vi "Test99.vi"(7 "L2T":T1 caption="Limites de test pris en compte", 8 "errin":errorcluster, 9 "SN":string="0B5MEVA000CA1JC1M0000041", 10 "OCV":string) -> (0 "errout":errorcluster, 2 "chaîne concaténée":string)   [LabVIEW 2020]
uses:
  <userlib>/Sylvain.lib/DATA_INSERT.vi
  VarGLO/Global var.vi
  Ctrl/L2T.ctl
panel:
  out "CMD":string
  in  "Cell 5 et 6":T2
  out "dataBDD":string[](array[string])
  in  "Cell 1 et 2":T2
  in  "Cell 3 et 4":T2
  out "Out":T3
  # "Pre DCIR_____________________________________"
  # "intra DCIR_____________________________________"
  # "Post DCIR_____________________________________"
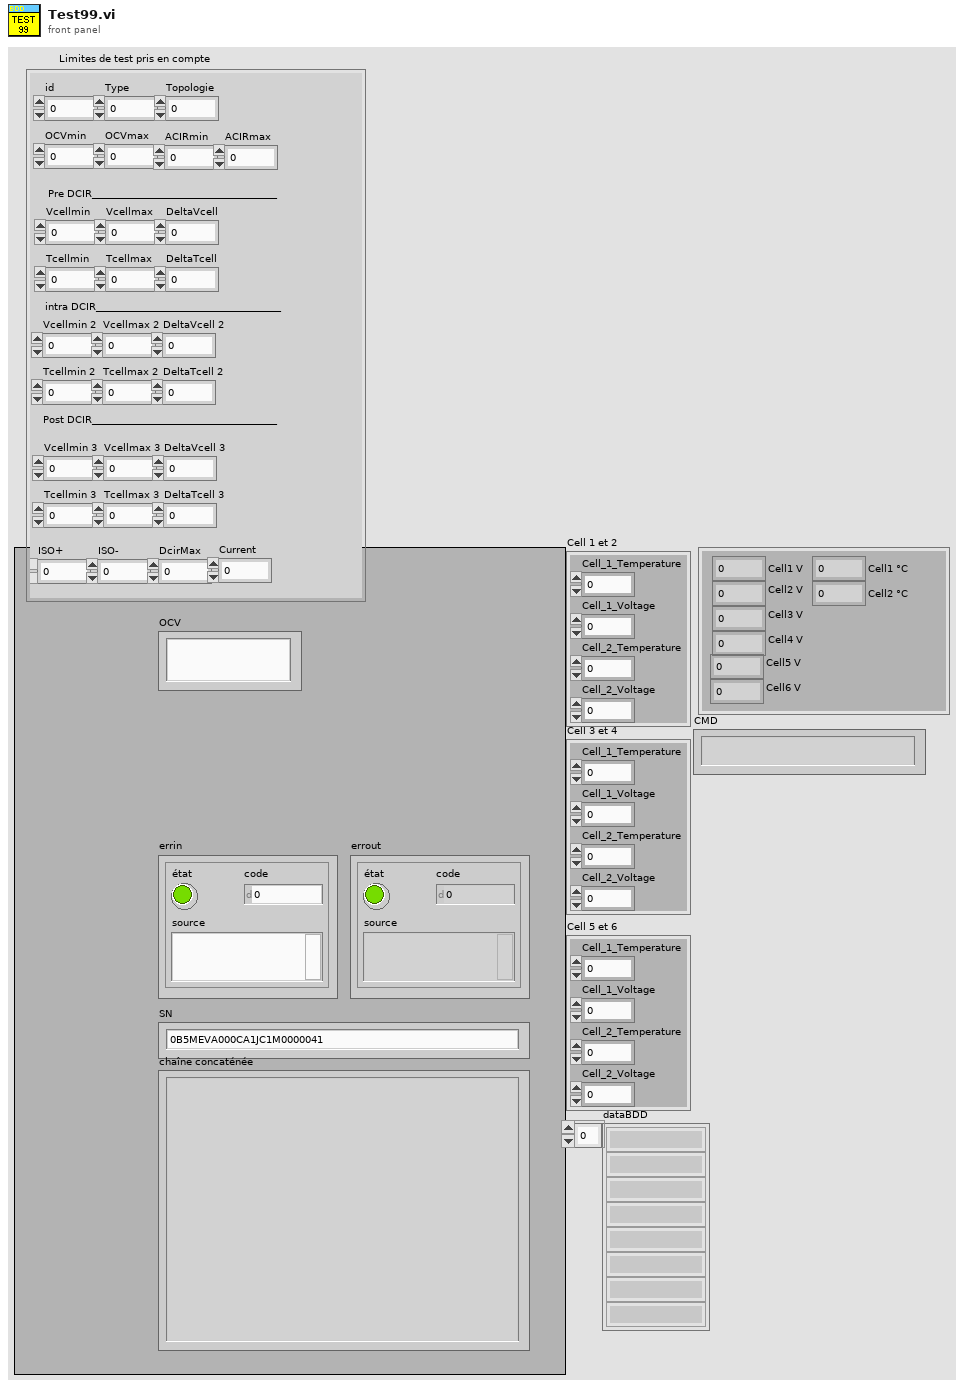
[diagram p1: front panel]
types:
  T1 = typedef "L2T.ctl" = cluster{"id":dbl, "Type":dbl, "OCVmin":dbl, "OCVmax":dbl, "ACIRmin":dbl, "ACIRmax":dbl, "Vcellmin":dbl, "Vcellmax":dbl, "DeltaVcell":dbl, "Tcellmin":dbl, "Tcellmax":dbl, "DeltaTcell":dbl, "ISO+":dbl, "ISO-":dbl, "DcirMax":dbl, "Current":dbl, "Topologie":dbl, "Vcellmin 2":dbl, "Vcellmax 2":dbl, "DeltaVcell 2":dbl, "Tcellmin 2":dbl, "Tcellmax 2":dbl, "DeltaTcell 2":dbl, "Vcellmin 3":dbl, "Vcellmax 3":dbl, "DeltaVcell 3":dbl, "Tcellmin 3":dbl, "Tcellmax 3":dbl, "DeltaTcell 3":dbl}
  T2 = cluster{"Cell_1_Temperature":sgl, "Cell_1_Voltage":sgl, "Cell_2_Temperature":sgl, "Cell_2_Voltage":sgl}
  T3 = cluster{"Cell1 V":sgl, "Cell2 V":sgl, "Cell3 V":sgl, "Cell4 V":sgl, "Cell1 °C":sgl, "Cell2 °C":sgl, "Cell5 V":sgl, "Cell6 V":sgl}
  T4 = cluster{"TempMin":sgl, "TempMax":sgl, "VoltageMin":sgl, "VoltageMax":sgl, "DeltaV":sgl, "DeltaC":sgl, "Ton":sgl}
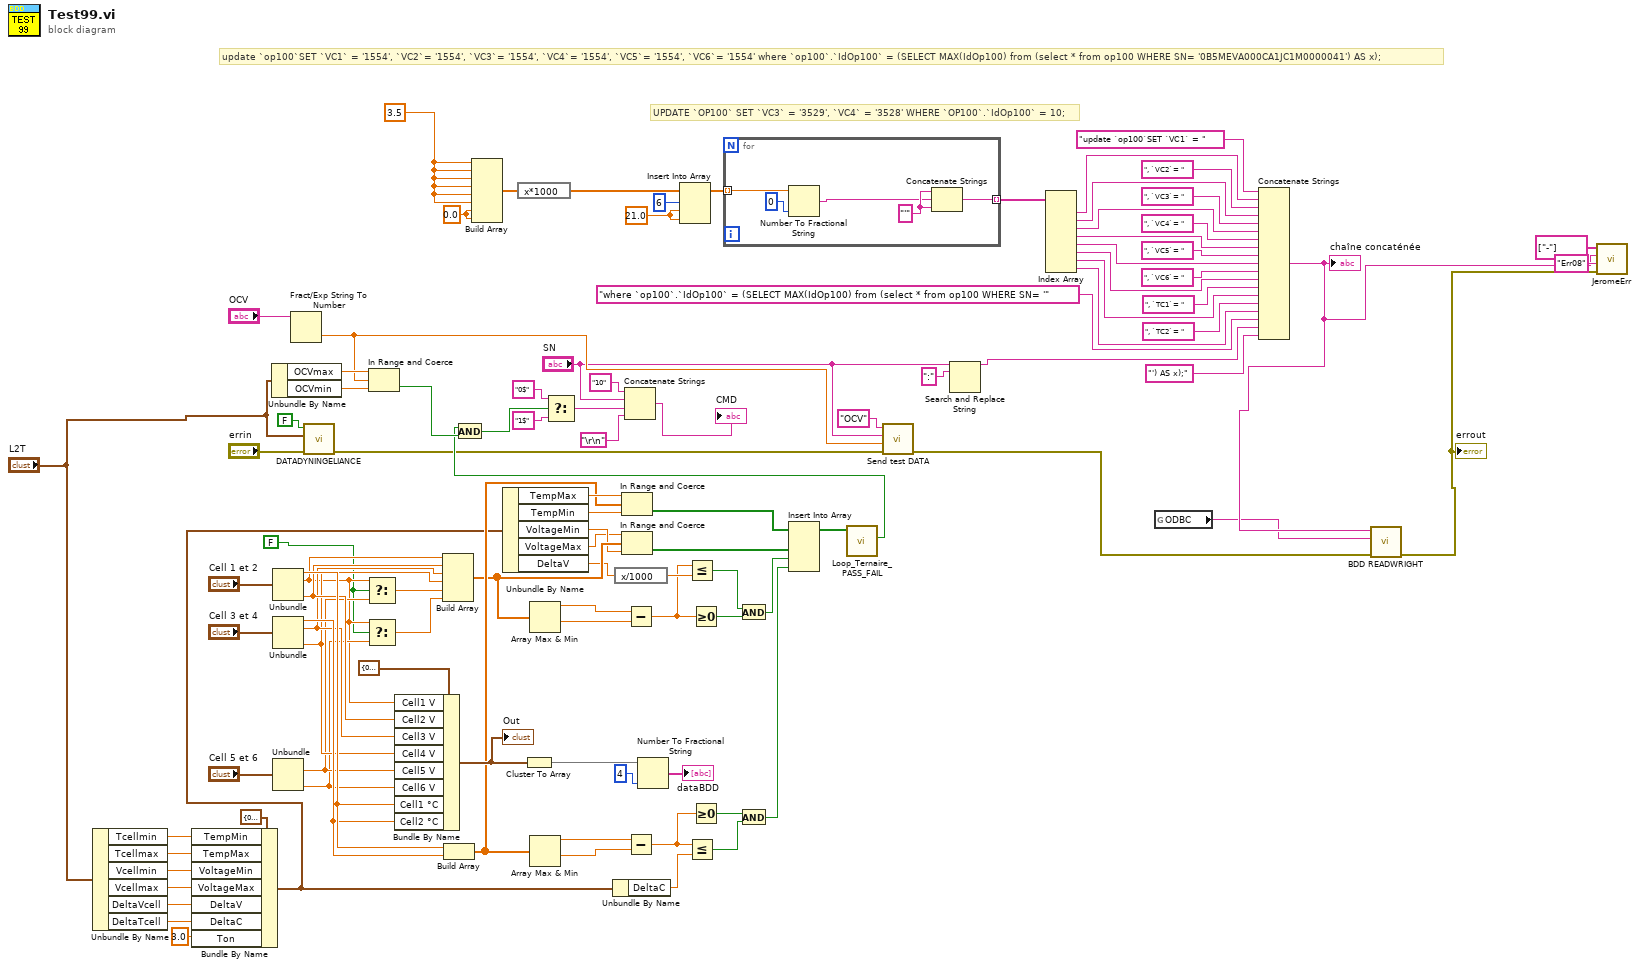
[diagram p0: block diagram]
diagram:
  w19 = FALSE ("sélecteur")
  w62 = sgl 21.0 ("nouvel élément/sous-tableau")
  w63 = sgl 3.5 ("élément")
  w99 = sgl 0.0 ("élément")
  # "update `op100`SET `VC1` = '1554', `VC2`= '1554', `VC3`= '1554', `VC4`= '1554', `VC5`= '1554', `VC6`= '1554' where `op100`.`IdOp100` = (SELECT MAX(IdOp100) from (select * from op100 WHERE SN= '0B5MEVA000CA1JC1M0000041') AS x);"
  # "UPDATE `OP100` SET `VC3` = '3529', `VC4` = '3528' WHERE `OP100`.`IdOp100` = 10;"
  n1 = Unbundle By Name("L2T") -> ("Tcellmin"=w17:dbl, "Tcellmax"=w16:dbl, "Vcellmin"=w15:dbl, "Vcellmax"=w14:dbl, "DeltaVcell"=w13:dbl, "DeltaTcell"=w12:dbl)
  n2 = Bundle By Name(cluster=T4 {"TempMin"=0.0, "TempMax"=0.0, "VoltageMin"=0.0, "VoltageMax"=0.0, "DeltaV"=0.0, "DeltaC"=0.0, "Ton"=0.0} ("Data out"), "TempMin"=w17, "TempMax"=w16, "VoltageMin"=w15, "VoltageMax"=w14, "DeltaV"=w13, "DeltaC"=w12, "Ton"=sgl 3.0) -> (w9:T4)
  n3 = Unbundle By Name("L2T") -> ("OCVmax"=w76:dbl, "OCVmin"=w75:dbl)
  n4 = Unbundle("Cell 1 et 2") -> ("Cell_1_Temperature"=w42:sgl, "Cell_1_Voltage"=w32:sgl, "Cell_2_Voltage"=w37:sgl)  [unwired: 1 out]
  n5 = Unbundle("Cell 3 et 4") -> ("Cell_1_Temperature"=w41:sgl, "Cell_1_Voltage"=w36:sgl, "Cell_2_Voltage"=w35:sgl)  [unwired: 1 out]
  n6 = Unbundle("Cell 5 et 6") -> ("Cell_1_Voltage"=w34:sgl, "Cell_2_Voltage"=w33:sgl)  [unwired: 2 out]
  n7 = Fract/Exp String To Number ("Chaîne Fract/Exp en nombre")(string="OCV") -> (number=w65:dbl)  [unwired: 3 in, 1 out]
  n8 = call "DATADYNINGELIANCE.vi"("errin"="errin", "L2T"="L2T", "3P4S"=FALSE) -> ("errout"=w8:errorcluster)  [unwired: 4 in, 4 out]
  n9 = Select(t=w32, s=w19, f=w34) -> (s? t:f=w31:sgl)
  n10 = Select(t=w32, s=w19, f=w33) -> (s? t:f=w30:sgl)
  n11 = In Range and Coerce(upper limit=w76, x=w65, lower limit=w75) -> (In Range?=w72:bool)  [unwired: 1 out]
  n12 = Bundle By Name(cluster=T3 {"Cell1 V"=0.0, "Cell2 V"=0.0, "Cell3 V"=0.0, "Cell4 V"=0.0, "Cell1 °C"=0.0, "Cell2 °C"=0.0, "Cell5 V"=0.0, "Cell6 V"=0.0} ("Out"), "Cell1 V"=w32, "Cell2 V"=w37, "Cell3 V"=w36, "Cell4 V"=w35, "Cell5 V"=w34, "Cell6 V"=w33, "Cell1 °C"=w42, "Cell2 °C"=w41) -> (w55:T3)
  "Out" <- w55
  n13 = Build Array(w32, w37, w36, w35, w31, w30) -> (w29:sgl[])
  n14 = Build Array(w42, w41) -> (w38:sgl[])
  n15 = Build Array(w63, w63, w63, w63, w63, w63, w99, w99) -> (w102:sgl[])
  n16 = Unbundle By Name(w9) -> ("TempMax"=w40:sgl, "TempMin"=w39:sgl, "VoltageMin"=w25:sgl, "VoltageMax"=w24:sgl, "DeltaV"=w26:sgl)
  n17 = expression code="x*1000"(w102) -> (w103:sgl[])
  n18 = Cluster To Array(cluster=w55) -> (array=w51:sgl[])
  n19 = Array Max & Min(array=w29) -> (max value=w47:sgl, min value=w46:sgl)  [unwired: 2 out]
  n20 = Array Max & Min(array=w38) -> (max value=w49:sgl, min value=w48:sgl)  [unwired: 2 out]
  n21 = Unbundle By Name(w9) -> ("DeltaC"=w28:sgl)
  n22 = expression code="x/1000"(w26) -> (w27:sgl)
  n23 = In Range and Coerce(upper limit=w40, x=w38, lower limit=w39) -> (In Range?=w54:bool[])  [unwired: 1 out]
  n24 = In Range and Coerce(upper limit=w24, x=w29, lower limit=w25) -> (In Range?=w53:bool[])  [unwired: 1 out]
  n25 = Subtract(x=w47, y=w46) -> (x-y=w20:sgl)
  n26 = Subtract(x=w49, y=w48) -> (x-y=w23:sgl)
  n27 = Number To Fractional String(number=w51, precision (6)=i16 4 ("précision (6)")) -> (F-format string=→"dataBDD":string[])  [unwired: 2 in]
  n28 = Insert Into Array(array=w103, index=6 ("indice"), new element #1=w62, new element #2=w62) -> (w105:sgl[])
  n29 = Less Or Equal?(x=w20, y=w27) -> (x <= y?=w44:bool)
  n30 = Less Or Equal?(x=w23, y=w28) -> (x <= y?=w45:bool)
  n31 = Greater Or Equal To 0?(x=w20) -> (x >= 0?=w21:bool)
  n32 = Greater Or Equal To 0?(x=w23) -> (x >= 0?=w22:bool)
  n33 = for {
    tunnel: w105 -> [w110] mode=indexing
    tunnel: [w107] -> w93 mode=indexing
    w108 = "'" ("chaîne")
    n34 = Number To Fractional String ("Nombre en chaîne fractionnaire")(number=w110, precision (6)=i16 0 ("précision (6)")) -> (F-format string=w106:string)  [unwired: 2 in]
    n35 = Concatenate Strings(w108, w106, w108) -> (w107:string)
  }
  n36 = And(x=w44, y=w21) -> (x .and. y?=w58:bool)
  n37 = And(x=w22, y=w45) -> (x .and. y?=w57:bool)
  n38 = Insert Into Array(array=w54, new element #1=w53, new element #2=w58, new element #3=w57) -> (w52:bool[])  [unwired: 1 in]
  n39 = call "Loop_Ternaire_PASS_FAIL.vi"("Tableau en entrée"=w52) -> ("ok global"=w18:bool)  [unwired: 9 in, 1 out]
  n40 = And(x=w18, y=w72) -> (x .and. y?=w71:bool)
  n41 = Select(t="0$" ("chaîne"), s=w71, f="1$" ("chaîne")) -> (s? t:f=w69:string)
  n42 = Concatenate Strings("10" ("chaîne"), "SN", w69, "\r\n") -> (→"CMD":string)
  n43 = call "Send test DATA.vi"("errin"=w8, "Value"=w65, "SN"="SN", "test"="OCV") -> ("error out"=w4:errorcluster)  [unwired: 7 in]
  n44 = Search and Replace String ("Rechercher et remplacer une chaîne")(input string="SN", search string=":" ("chaîne recherchée")) -> (result string=w95:string)  [unwired: 6 in, 3 out]
  n45 = Index Array(array=w93) -> (element #1=w92:string, element #2=w90:string, element #3=w88:string, element #4=w86:string, element #5=w84:string, element #6=w82:string, element #7=w81:string, element #8=w78:string)  [unwired: 8 in]
  n46 = global read "Global var.vi" "ODBC"() -> (w1:string)
  n47 = Concatenate Strings("update `op100`SET `VC1` = " ("chaîne"), w92, ", `VC2`= " ("chaîne"), w90, ", `VC3`= " ("chaîne"), w88, ", `VC4`= " ("chaîne"), w86, ", `VC5`= " ("chaîne"), w84, ", `VC6`= " ("chaîne"), w82, ", `TC1`= " ("chaîne"), w81, ", `TC2`= " ("chaîne"), w78, "where `op100`.`IdOp100` = (SELECT MAX(IdOp100) from (select * from op100 WHERE SN= '" ("chaîne"), w95, "') AS x);" ("chaîne")) -> (w3:string)
  "chaîne concaténée" <- w3
  n48 = call "BDD READWRIGHT.vi"("errin"=w4, 10:w1, "INSERT"=w3) -> ("errout"=w2:errorcluster)  [unwired: 8 in]
  "errout" <- w2
  n49 = call "JeromeErr.vi"("Errin"=w2, "CodeERR"="Err08", "RequetteSQL"=w3, "RetourSQL"=string[] ["-"]) -> ()  [unwired: 8 in]
